vi "E4981_command.vi"(8 "error in (no error)":errorcluster, 10 "input":T1={"Frequency (1:1kHz)"=1, "Frequency Shift (2: 0%)"=2, "Range"=enum."1p"} {"Frequency Shift (2: 0%)" items=["-2%", "-1%", "0%", "1%", "2%"]; "Frequency (1:1kHz)" items=["120 Hz Frequency", "1 kHz Frequency", "1 MHz Frequency"]}, 11 "command":T3(ring)) -> (0 "error out":errorcluster, 1 "bin":i32, 3 "output":T2={"connectd"=TRUE, "CAP cab"=0.0, "DF  Cab"=0.0} {"CAP cab" format="%#_6p"})   [LabVIEW 2016]
uses:
  meter global.vi
  AOIFramwork/AOIFramework.lvlib
panel:
  in  "reset":bool
  # "CAP DF 電錶作業中"
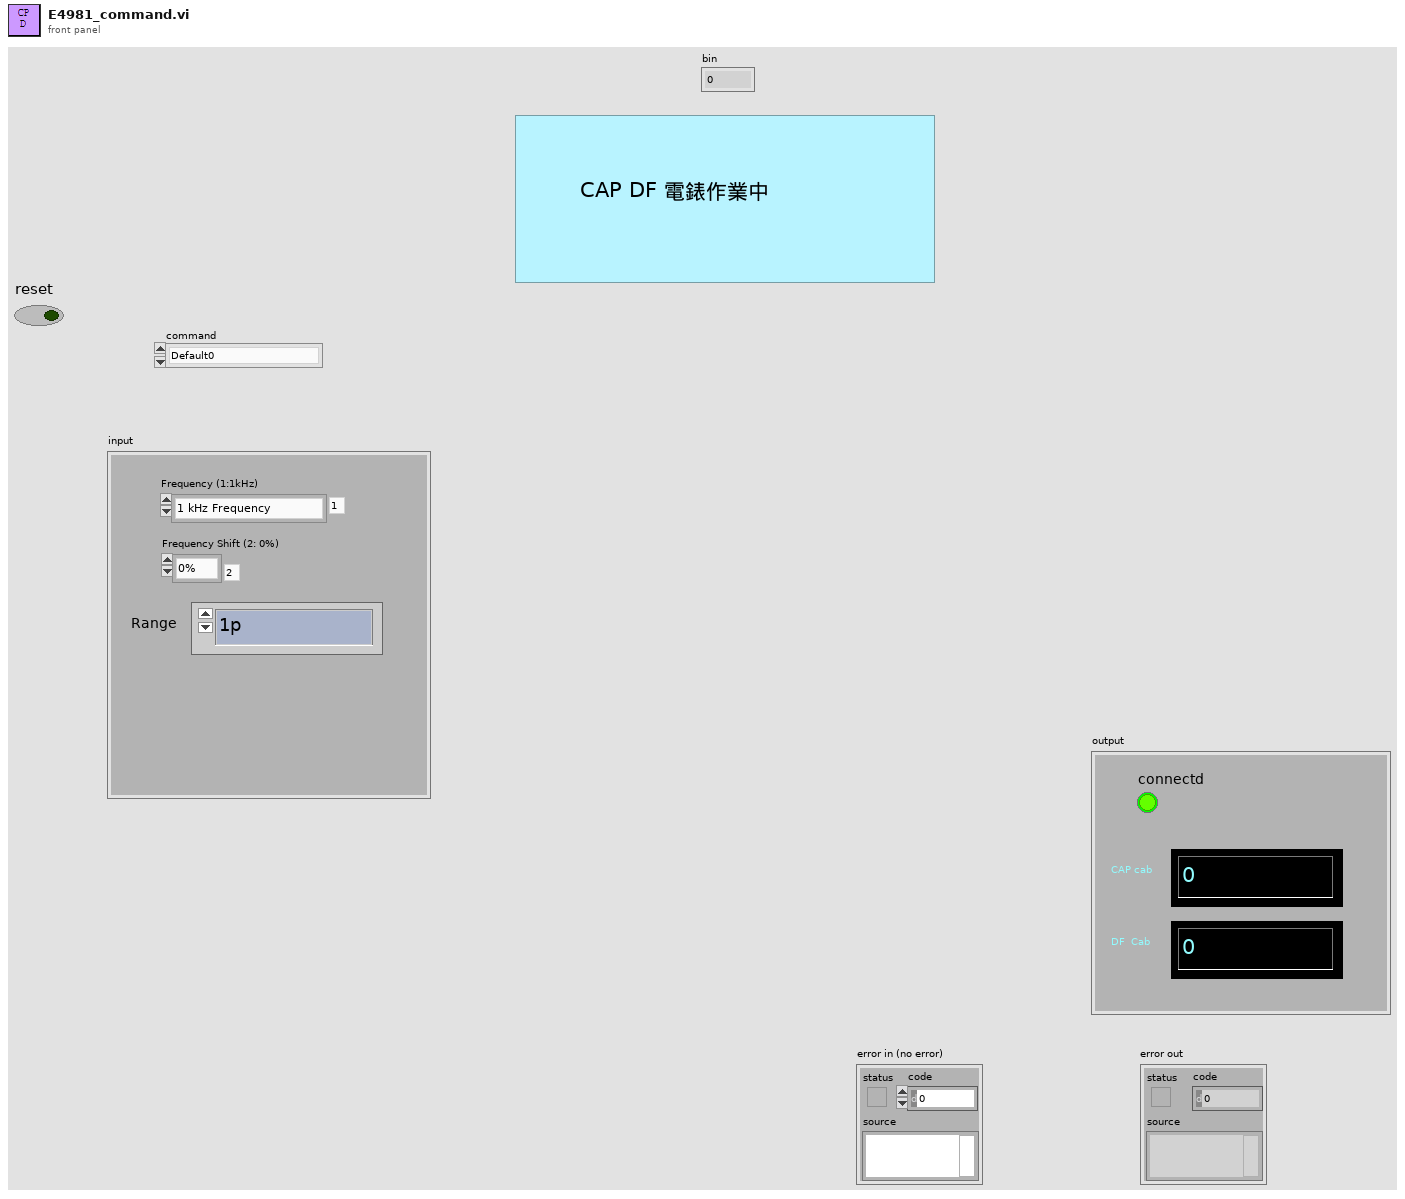
[diagram p1: front panel]
types:
  T1 = cluster{"Frequency (1:1kHz)":u16, "Frequency Shift (2: 0%)":u16, "Range":enum16{"1p", "2.2p", "4.7p", "10p", "22p", "47p", "100p", "220p", "470p", "1n", "2.2n", "4.7n", "10n", "22n", "47n", "100n", "220n", "470n", "1u", "2.2u", "4.7u", "10u", "22u", "47u", "100u", "220u", "470u", "1m", "AUTO", ""}}
  T2 = cluster{"connectd":bool, "CAP cab":dbl, "DF  Cab":dbl}
  T3 = enum16{"Default0", "checkconnect", "int", "changeFEQ", "changeRange", "trigger", "triggerauto"}
  T4 = enum16{"1p", "2.2p", "4.7p", "10p", "22p", "47p", "100p", "220p", "470p", "1n", "2.2n", "4.7n", "10n", "22n", "47n", "100n", "220n", "470n", "1u", "2.2u", "4.7u", "10u", "22u", "47u", "100u", "220u", "470u", "1m", "AUTO", ""}
  T5 = typedef "TypeDef_PNData.ctl" = cluster{"External Diameter":dbl, "Height":dbl, "Range":enum16{"1p", "2.2p", "4.7p", "10p", "22p", "47p", "100p", "220p", "470p", "1n", "2.2n", "4.7n", "10n", "22n", "47n", "100n", "220n", "470n", "1u", "2.2u", "4.7u", "10u", "22u", "47u", "100u", "220u", "470u", "1m", "AUTO", ""}, "DFmin":dbl, "Cap_num":dbl, "F":u16, "BIN3+":dbl, "BIN3- ":dbl, "BIN2+":dbl, "BIN2-":dbl, "BIN1+":dbl, "BIN1-":dbl, "Frequencies":enum16{"120HZ", "1K  HZ", "1M HZ"}, "DFmax":dbl, "Part_5":dbl, "Part_6":dbl, "Part_4":dbl, "Part_8":dbl, "Part_7":dbl, "Par_2":dbl, "part_1":enum16{"DC", "AC"}, "Part_9":dbl, "Part_18":dbl, "Part_15":dbl, "Part_13":dbl, "Part_14":dbl, "Part_16":dbl, "Internal Diameter":dbl, "Part_14 (IR Max)":dbl, "SCARA Place Offset":T6}
  T6 = typedef "MachineParTypeSCARA PlaceOffset.ctl" = cluster{"Buffer":cluster{"X":dbl, "Y":dbl, "Z":dbl}, "UNLD":cluster{"X":dbl, "Y":dbl, "Z":dbl}}
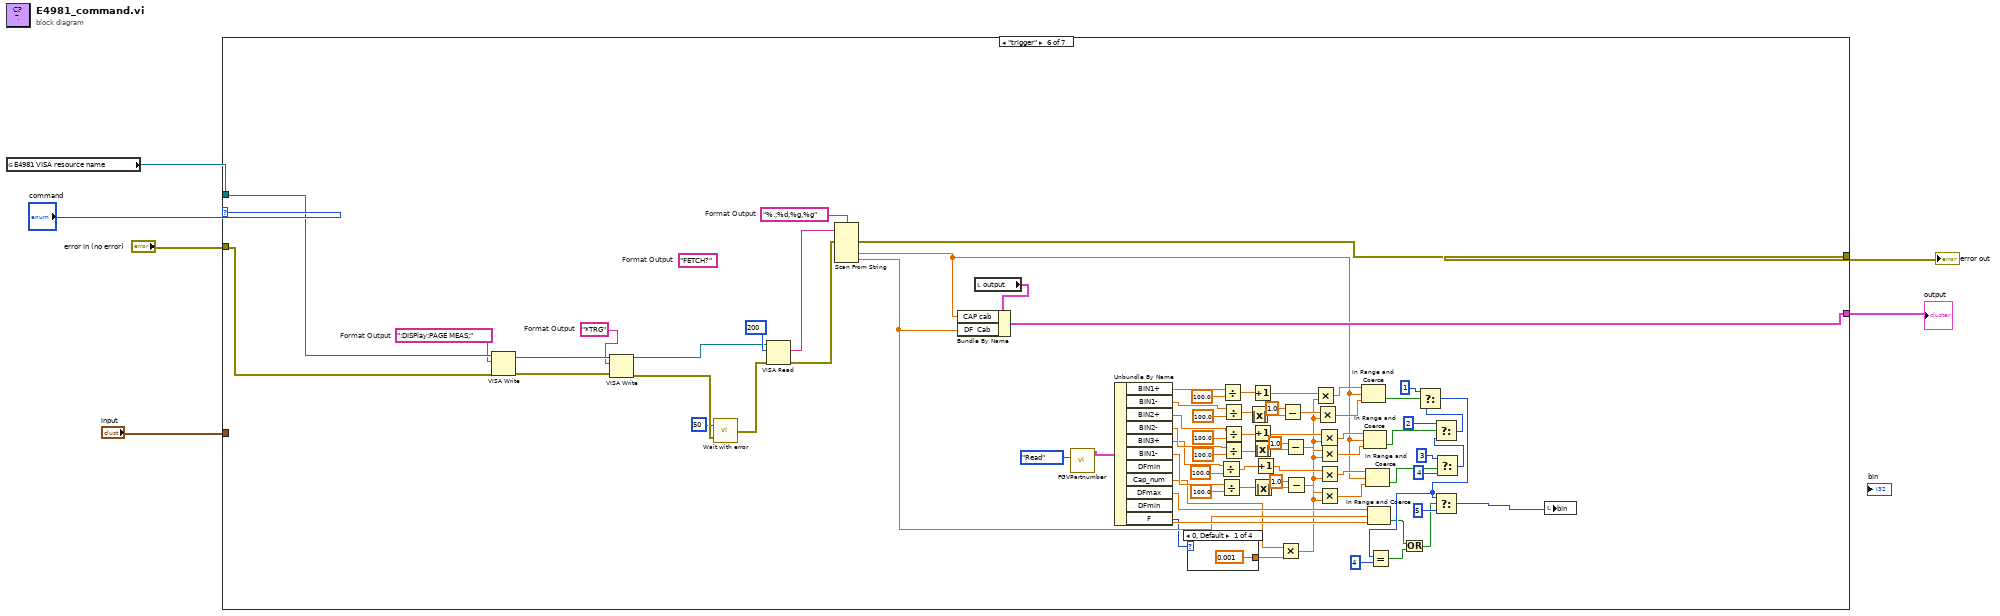
[diagram p0: block diagram]
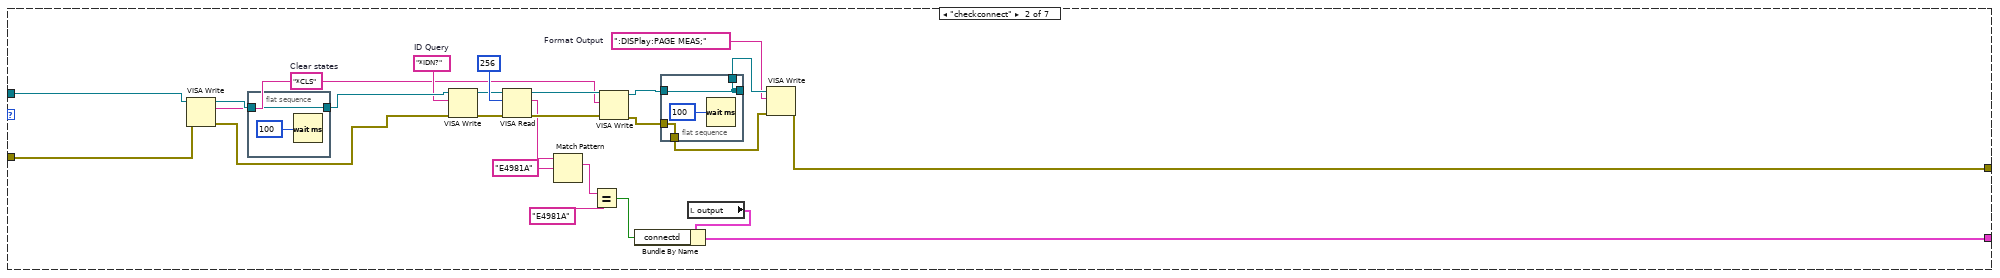
[diagram p3: hidden frame]
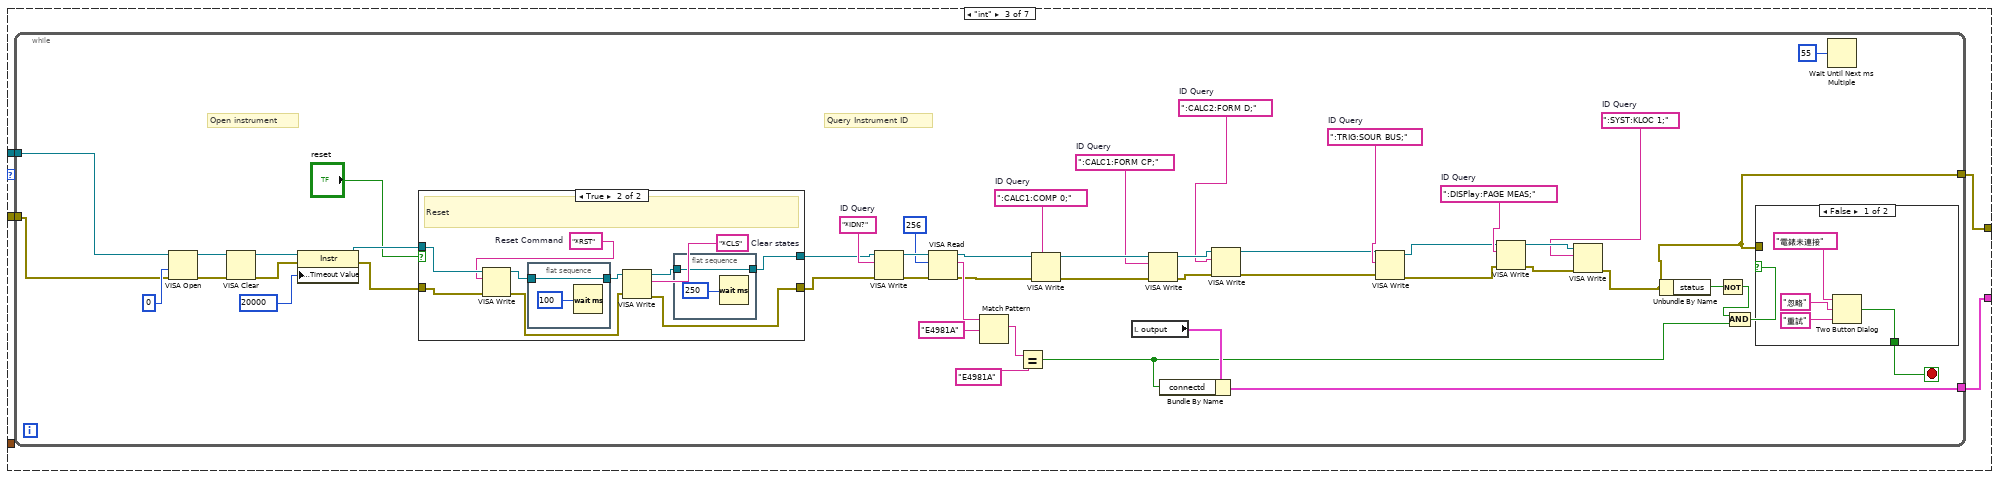
[diagram p4: hidden frame]
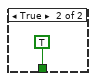
[diagram p6: hidden frame]
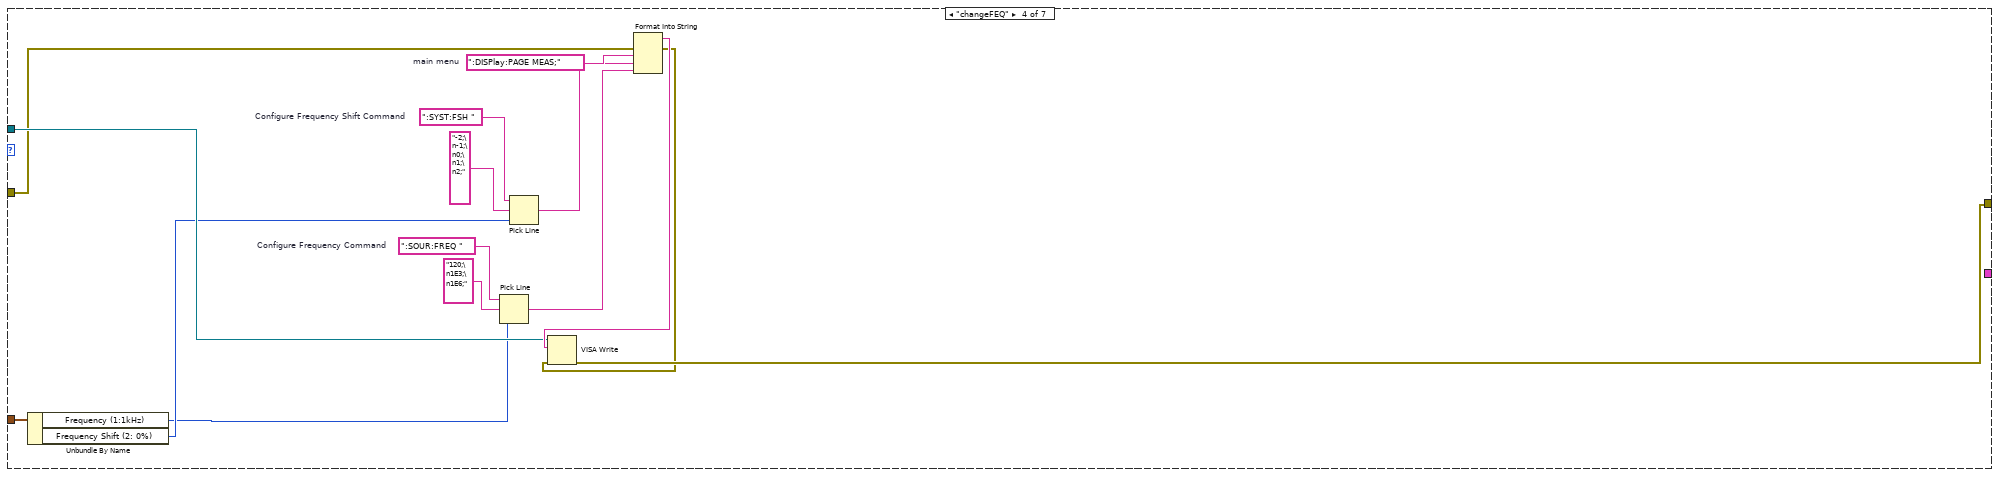
[diagram p7: hidden frame]
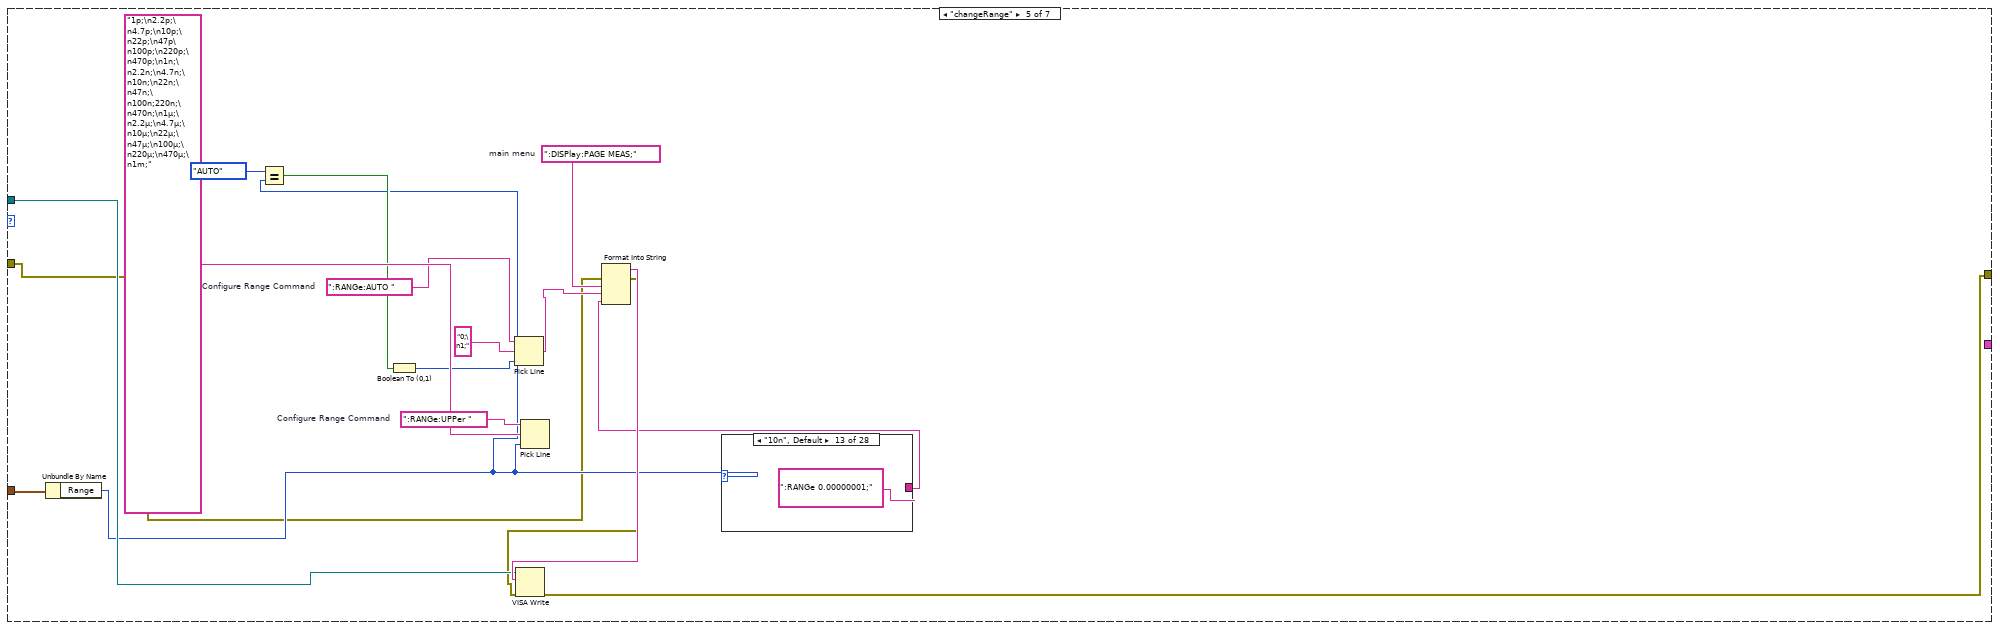
[diagram p8: hidden frame]
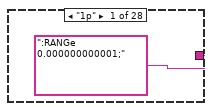
[diagram p9: hidden frame]
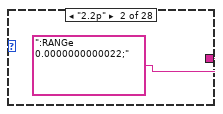
[diagram p10: hidden frame]
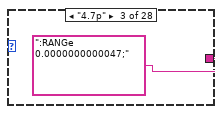
[diagram p11: hidden frame]
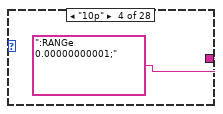
[diagram p12: hidden frame]
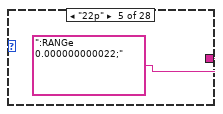
[diagram p13: hidden frame]
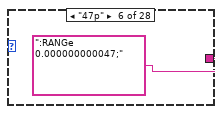
[diagram p14: hidden frame]
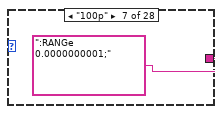
[diagram p15: hidden frame]
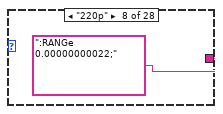
[diagram p16: hidden frame]
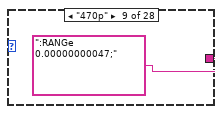
[diagram p17: hidden frame]
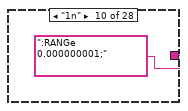
[diagram p18: hidden frame]
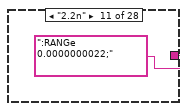
[diagram p19: hidden frame]
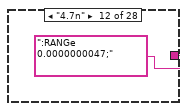
[diagram p20: hidden frame]
diagram:
  n1 = global read "meter global.vi" "E4981 VISA resource name"() -> (w4:refnum<visa-resource-name>)
  n2 = case shown="\"trigger\"" "command" {
    tunnel: "error in (no error)" -> [_ w13 w38 w111 w126 w240 w319]
    tunnel: [_ w12 w40 w115 w129 w235 w261] -> w5
    tunnel: w4 -> [_ w10 w39 w116 w130 w241 w320]
    tunnel: [_ w7 w37 _ _ w238 w317] -> w2
    tunnel: "input" -> [_ _ _ w114 w128 _ _]
    frame "Default0", Default {
    }
    frame "checkconnect" {
      w27 = ":DISPlay:PAGE MEAS;"  # Format Output
      w11 = "*CLS"  # Clear states
      w19 = "*IDN?"  # ID Query
      n3 = VISA Write(VISA resource name=w10, write buffer=w11, error in (no error)=w13) -> (VISA resource name out=w24:refnum<visa-resource-name>, error out=w23:errorcluster)  [unwired: 1 out]
      n4 = flat-sequence {
        tunnel: [w35] -> w22
        tunnel: w24 -> [w35]
        frame #0 {
          n5 = Wait (ms)(milliseconds to wait=u32 100) -> ()  [unwired: 1 out]
        }
      }
      n6 = VISA Write(VISA resource name=w22, write buffer=w19, error in (no error)=w23) -> (VISA resource name out=w15:refnum<visa-resource-name>, error out=w16:errorcluster)  [unwired: 1 out]
      n7 = VISA Read(VISA resource name=w15, byte count=u32 256, error in (no error)=w16) -> (VISA resource name out=w25:refnum<visa-resource-name>, read buffer=w14:string, error out=w26:errorcluster)  [unwired: 1 out]
      n8 = Match Pattern(string=w14, regular expression="E4981A") -> (match substring=w20:string)  [unwired: 1 in, 3 out]
      n9 = Equal?(x=w20, y="E4981A") -> (x = y?=w8:bool)
      n10 = VISA Write(VISA resource name=w25, write buffer=w11, error in (no error)=w26) -> (VISA resource name out=w28:refnum<visa-resource-name>, error out=w29:errorcluster)  [unwired: 1 out]
      n11 = flat-sequence {
        tunnel: [w32] -> _
        tunnel: w28 -> [w32]
        tunnel: w29 -> [w33]
        tunnel: [w33] -> w30
        tunnel: [w32] -> w31
        frame #0 {
          n12 = Wait (ms)(milliseconds to wait=u32 100) -> ()  [unwired: 1 out]
        }
      }
      n13 = local read "output"() -> (w9:T2)
      n14 = Bundle By Name(cluster=w9, "connectd"=w8) -> (w7:T2)
      n15 = VISA Write(VISA resource name=w31, write buffer=w27, error in (no error)=w30) -> (error out=w12:errorcluster)  [unwired: 2 out]
    }
    frame "int" {
      n16 = while {
        tunnel: [w46] -> w40
        tunnel: w39 -> [w45]
        tunnel: w38 -> [w44]
        tunnel: [w41] -> w37
        stop <- w73 stop-if-true
        w54 = ":TRIG:SOUR BUS;"  # ID Query
        w57 = ":SYST:KLOC 1;"  # ID Query
        w60 = ":DISPlay:PAGE MEAS;"  # ID Query
        w61 = ":CALC2:FORM D;"  # ID Query
        w62 = ":CALC1:FORM CP;"  # ID Query
        w71 = ":CALC1:COMP 0;"  # ID Query
        w77 = "*IDN?"  # ID Query
        # "Query Instrument ID"
        # "Open instrument"
        n17 = VISA Open(access mode=u32 0, error in (no error)=w44, VISA resource name=w45) -> (VISA resource name=w86:refnum<visa-resource-name>, error out=w85:errorcluster)  [unwired: 2 in]
        n18 = VISA Clear(VISA resource name=w86, error in (no error)=w85) -> (VISA resource name out=w84:refnum<visa-resource-name>, error out=w83:errorcluster)
        n19 = property class="Instr"(reference=w84, error in=w83, "General Settings:Timeout Value"=u32 20000) -> (reference out=w50:refnum<visa-resource-name>, error out=w48:errorcluster)
        n20 = case shown="True" "reset" {
          tunnel: [w90 w95] -> w51
          tunnel: w50 -> [w90 w100]
          tunnel: [w89 w93] -> w49
          tunnel: w48 -> [w89 w92]
          frame False {
          }
          frame True {
            w91 = "*CLS"  # Clear states
            w99 = "*RST"  # Reset Command
            # "Reset"
            n21 = VISA Write(VISA resource name=w100, write buffer=w99, error in (no error)=w92) -> (VISA resource name out=w97:refnum<visa-resource-name>, error out=w94:errorcluster)  [unwired: 1 out]
            n22 = flat-sequence {
              tunnel: [w103] -> w98
              tunnel: w97 -> [w103]
              frame #0 {
                n23 = Wait (ms)(milliseconds to wait=u32 100) -> ()  [unwired: 1 out]
              }
            }
            n24 = VISA Write(VISA resource name=w98, write buffer=w91, error in (no error)=w94) -> (VISA resource name out=w96:refnum<visa-resource-name>, error out=w93:errorcluster)  [unwired: 1 out]
            n25 = flat-sequence {
              tunnel: [w101] -> w95
              tunnel: w96 -> [w101]
              frame #0 {
                n26 = Wait (ms)(milliseconds to wait=u32 250) -> ()  [unwired: 1 out]
              }
            }
          }
        }
        n27 = VISA Write(VISA resource name=w51, write buffer=w77, error in (no error)=w49) -> (VISA resource name out=w81:refnum<visa-resource-name>, error out=w80:errorcluster)  [unwired: 1 out]
        n28 = VISA Read(VISA resource name=w81, byte count=u32 256, error in (no error)=w80) -> (VISA resource name out=w69:refnum<visa-resource-name>, read buffer=w82:string, error out=w70:errorcluster)  [unwired: 1 out]
        n29 = Match Pattern(string=w82, regular expression="E4981A") -> (match substring=w75:string)  [unwired: 1 in, 3 out]
        n30 = Equal?(x=w75, y="E4981A") -> (x = y?=w42:bool)
        n31 = VISA Write(VISA resource name=w69, write buffer=w71, error in (no error)=w70) -> (VISA resource name out=w66:refnum<visa-resource-name>, error out=w65:errorcluster)  [unwired: 1 out]
        n32 = local read "output"() -> (w43:T2)
        n33 = VISA Write(VISA resource name=w66, write buffer=w62, error in (no error)=w65) -> (VISA resource name out=w63:refnum<visa-resource-name>, error out=w64:errorcluster)  [unwired: 1 out]
        n34 = Bundle By Name(cluster=w43, "connectd"=w42) -> (w41:T2)
        n35 = VISA Write(VISA resource name=w63, write buffer=w61, error in (no error)=w64) -> (VISA resource name out=w53:refnum<visa-resource-name>, error out=w52:errorcluster)  [unwired: 1 out]
        n36 = VISA Write(VISA resource name=w53, write buffer=w54, error in (no error)=w52) -> (VISA resource name out=w56:refnum<visa-resource-name>, error out=w55:errorcluster)  [unwired: 1 out]
        n37 = VISA Write(VISA resource name=w56, write buffer=w60, error in (no error)=w55) -> (VISA resource name out=w58:refnum<visa-resource-name>, error out=w59:errorcluster)  [unwired: 1 out]
        n38 = VISA Write(VISA resource name=w58, write buffer=w57, error in (no error)=w59) -> (error out=w46:errorcluster)  [unwired: 2 out]
        n39 = Unbundle By Name(w46) -> ("status"=w68:bool)
        n40 = Not(x=w68) -> (.not. x?=w67:bool)
        n41 = And(x=w67, y=w42) -> (x .and. y?=w76:bool)
        n42 = case shown="False" w76 {
          tunnel: [w107 TRUE ("cancel 2")] -> w73
          tunnel: w46 -> [_ _]
          frame False {
            n43 = Two Button Dialog(message="電錶未連接", 1:"重試" ("T button name (\"OK\")"), 2:"忽略" ("F button name (\"Cancel\")")) -> (T button?=w107:bool)
          }
          frame True {
          }
        }
        n44 = Wait Until Next ms Multiple(millisecond multiple=u32 55) -> ()  [unwired: 1 out]
      }
    }
    frame "changeFEQ" {
      w120 = ":DISPlay:PAGE MEAS;"  # main menu
      w121 = ":SYST:FSH "  # Configure Frequency Shift Command
      w122 = ":SOUR:FREQ "  # Configure Frequency Command
      n45 = Unbundle By Name(w114) -> ("Frequency (1:1kHz)"=w112:u16, "Frequency Shift (2: 0%)"=w113:u16)
      n46 = Pick Line(string ("")=w122, multi-line string="120;\n1E3;\n1E6;", line index=w112) -> (output string=w118:string)
      n47 = Pick Line(string ("")=w121, multi-line string="-2;\n-1;\n0;\n1;\n2;", line index=w113) -> (output string=w119:string)
      n48 = Format Into String(error in=w111, w120, w119, w118) -> (resulting string=w117:string, error out=w110:errorcluster)  [unwired: 2 in]
      n49 = VISA Write(VISA resource name=w116, write buffer=w117, error in (no error)=w110) -> (error out=w115:errorcluster)  [unwired: 2 out]
    }
    frame "changeRange" {
      w139 = ":RANGe:UPPer "  # Configure Range Command
      w136 = ":RANGe:AUTO "  # Configure Range Command
      w141 = ":DISPlay:PAGE MEAS;"  # main menu
      n50 = Unbundle By Name(w128) -> ("Range"=w127:T4)
      n51 = Equal?(x=T4."AUTO", y=w127) -> (x = y?=w134:bool)
      n52 = Boolean To (0,1)(Boolean=w134) -> (0, 1=w133:i16)
      n53 = Pick Line(string ("")=w136, multi-line string="0;\n1;", line index=w133) -> (output string=w132:string)
      n54 = Pick Line(string ("")=w139, multi-line string="1p;\n2.2p;\n4.7p;\n10p;\n22p;\n47p\n100p;\n220p;\n470p;\n1n;\n2.2n;\n4.7n;\n10n;\n22n;\n47n;\n100n;220n;\n470n;\n1μ;\n2.2μ;\n4.7μ;\n10μ;\n22μ;\n47μ;\n100μ;\n220μ;\n470μ;\n1m;", line index=w127) -> ()  [unwired: 1 out]
      n55 = case shown="\"10n\", Default" w127 {
        tunnel: [":RANGe 0.000000000001;" ("Configure Range Command") ":RANGe 0.0000000000022;" ("Configure Range Command") ":RANGe 0.0000000000047;" ("Configure Range Command") ":RANGe 0.00000000001;" ("Configure Range Command") ":RANGe 0.000000000022;" ("Configure Range Command") ":RANGe 0.000000000047;" ("Configure Range Command") ":RANGe 0.0000000001;" ("Configure Range Command") ":RANGe 0.00000000022;" ("Configure Range Command") ":RANGe 0.00000000047;" ("Configure Range Command") ":RANGe 0.000000001;" ("Configure Range Command") ":RANGe 0.0000000022;" ("Configure Range Command") ":RANGe 0.0000000047;" ("Configure Range Command") ":RANGe 0.00000001;" ("Configure Range Command") ":RANGe 0.000000022;" ("Configure Range Command") ":RANGe 0.000000047;" ("Configure Range Command") ":RANGe 0.0000001;" ("Configure Range Command") ":RANGe 0.00000022;" ("Configure Range Command") ":RANGe 0.00000047;" ("Configure Range Command") ":RANGe 0.000001;" ("Configure Range Command") ":RANGe 0.0000022;" ("Configure Range Command") ":RANGe 0.0000047;" ("Configure Range Command") ":RANGe 0.00001;" ("Configure Range Command") ":RANGe 0.000022;" ("Configure Range Command") ":RANGe 0.000047;" ("Configure Range Command") ":RANGe 0.0001;" ("Configure Range Command") ":RANGe 0.00022;" ("Configure Range Command") ":RANGe 0.00047;" ("Configure Range Command") ":RANGe 0.001;" ("Configure Range Command")] -> w131
        frame "1p" {
        }
        frame "2.2p" {
        }
        frame "4.7p" {
        }
        frame "10p" {
        }
        frame "22p" {
        }
        frame "47p" {
        }
        frame "100p" {
        }
        frame "220p" {
        }
        frame "470p" {
        }
        frame "1n" {
        }
        frame "2.2n" {
        }
        frame "4.7n" {
        }
        frame "10n", Default {
        }
        frame "22n" {
        }
        frame "47n" {
        }
        frame "100n" {
        }
        frame "220n" {
        }
        frame "470n" {
        }
        frame "1u" {
        }
        frame "2.2u" {
        }
        frame "4.7u" {
        }
        frame "10u" {
        }
        frame "22u" {
        }
        frame "47u" {
        }
        frame "100u" {
        }
        frame "220u" {
        }
        frame "470u" {
        }
        frame "1m" {
        }
      }
      n56 = Format Into String(error in=w126, w141, w132, w131) -> (resulting string=w140:string, error out=w125:errorcluster)  [unwired: 2 in]
      n57 = VISA Write(VISA resource name=w130, write buffer=w140, error in (no error)=w125) -> (error out=w129:errorcluster)  [unwired: 2 out]
    }
    frame "trigger" {
      w237 = ":DISPlay:PAGE MEAS;"  # Format Output
      (unwired) "FETCH?"  # Format Output
      w242 = "*TRG"  # Format Output
      w246 = "%.;%d,%g,%g"  # Format Output
      n58 = VISA Write(VISA resource name=w241, write buffer=w237, error in (no error)=w240) -> (VISA resource name out=w243:refnum<visa-resource-name>, error out=w244:errorcluster)  [unwired: 1 out]
      n59 = VISA Write(VISA resource name=w243, write buffer=w242, error in (no error)=w244) -> (VISA resource name out=w245:refnum<visa-resource-name>, error out=w177:errorcluster)  [unwired: 1 out]
      n60 = call "Wait with error.vi"("error in (no error)"=w177, "milliseconds to wait"=u32 50) -> ("error out"=w176:errorcluster)
      n61 = VISA Read(VISA resource name=w245, byte count=u32 200, error in (no error)=w176) -> (read buffer=w247:string, error out=w236:errorcluster)  [unwired: 2 out]
      n62 = Scan From String(format string=w246, input string=w247, error in=w236) -> (error out=w235:errorcluster, output 2=w183:dbl, output 3=w182:dbl)  [unwired: 5 in, 2 out]
      n63 = local read "output"() -> (w239:T2)
      n64 = Bundle By Name(cluster=w239, "CAP cab"=w183, "DF  Cab"=w182) -> (w238:T2)
      n65 = call "FGVPartnumber.vi"("Enum"=enum16{"Write", "Read"}."Read") -> ("UnitParamiterCluster out"=w233:T5)  [unwired: 9 in, 1 out]
      n66 = Unbundle By Name(w233) -> ("BIN1+"=w232:dbl, "BIN1-"=w229:dbl, "BIN2+"=w227:dbl, "BIN2-"=w225:dbl, "BIN3+"=w223:dbl, "BIN1-"=w221:dbl, "Cap_num"=w179:dbl, "DFmax"=w196:dbl, "DFmin"=w195:dbl, "F"=w181:u16)  [unwired: 1 out]
      n67 = case shown="0, Default" w181 {
        tunnel: [0.001 1e-06 1e-09 1e-12] -> w180
        frame 0, Default {
        }
        frame 1 {
        }
        frame 2 {
        }
        frame 3 {
        }
      }
      n68 = Divide(x=w223, y=100.0) -> (x/y=w209:dbl)
      n69 = Divide(x=w221, y=100.0) -> (x/y=w211:dbl)
      n70 = Divide(x=w232, y=100.0) -> (x/y=w220:dbl)
      n71 = Divide(x=w229, y=100.0) -> (x/y=w219:dbl)
      n72 = Divide(x=w227, y=100.0) -> (x/y=w210:dbl)
      n73 = Divide(x=w225, y=100.0) -> (x/y=w214:dbl)
      n74 = Absolute Value(x=w219) -> (abs(x)=w218:dbl)
      n75 = Increment(x=w220) -> (x+1=w208:dbl)
      n76 = Increment(x=w210) -> (x+1=w206:dbl)
      n77 = Absolute Value(x=w214) -> (abs(x)=w215:dbl)
      n78 = Absolute Value(x=w211) -> (abs(x)=w213:dbl)
      n79 = Increment(x=w209) -> (x+1=w204:dbl)
      n80 = Multiply(x=w179, y=w180) -> (x*y=w178:dbl)
      n81 = Subtract(x=1.0, y=w218) -> (x-y=w207:dbl)
      n82 = Subtract(x=1.0, y=w215) -> (x-y=w205:dbl)
      n83 = Subtract(x=1.0, y=w213) -> (x-y=w203:dbl)
      n84 = Multiply(x=w208, y=w178) -> (x*y=w202:dbl)
      n85 = Multiply(x=w207, y=w178) -> (x*y=w201:dbl)
      n86 = Multiply(x=w206, y=w178) -> (x*y=w200:dbl)
      n87 = Multiply(x=w205, y=w178) -> (x*y=w199:dbl)
      n88 = Multiply(x=w204, y=w178) -> (x*y=w198:dbl)
      n89 = Multiply(x=w203, y=w178) -> (x*y=w197:dbl)
      n90 = In Range and Coerce(upper limit=w202, x=w183, lower limit=w201) -> (In Range?=w194:bool)  [unwired: 1 out]
      n91 = In Range and Coerce(upper limit=w200, x=w183, lower limit=w199) -> (In Range?=w187:bool)  [unwired: 1 out]
      n92 = In Range and Coerce(upper limit=w198, x=w183, lower limit=w197) -> (In Range?=w189:bool)  [unwired: 1 out]
      n93 = In Range and Coerce(upper limit=w196, x=w182, lower limit=w195) -> (In Range?=w171:bool)  [unwired: 1 out]
      n94 = Select(t=3, s=w189, f=4) -> (s? t:f=w188:i32)
      n95 = Select(t=2, s=w187, f=w188) -> (s? t:f=w186:i32)
      n96 = Select(t=1, s=w194, f=w186) -> (s? t:f=w174:i32)
      n97 = Equal?(x=w174, y=4) -> (x = y?=w172:bool)
      n98 = Or(x=w171, y=w172) -> (x .or. y?=w170:bool)
      n99 = Select(t=w174, s=w170, f=5) -> (s? t:f=w184:i32)
      n100 = local write "bin"(w184) -> ()
    }
    frame "triggerauto" {
      w316 = enum16{"Write", "Read"}."Read"  # Enum
      (unwired) "FETCH?"  # Format Output
      w321 = "*TRG"  # Format Output
      w325 = "%.;%d,%g,%g"  # Format Output
      n101 = disable-structure shown="Disabled" {
        disable-tunnel: [w336 w337] -> w323
        disable-tunnel: [w335 w338] -> w322
        disable-tunnel: w320 -> [w334 w338]
        disable-tunnel: w319 -> [w333 w337]
        frame Disabled {
          w332 = ":DISPlay:PAGE MEAS;"  # Format Output
          n102 = VISA Write(VISA resource name=w334, write buffer=w332, error in (no error)=w333) -> (VISA resource name out=w335:refnum<visa-resource-name>, error out=w336:errorcluster)  [unwired: 1 out]
        }
        frame Enabled {
        }
      }
      n103 = VISA Write(VISA resource name=w322, write buffer=w321, error in (no error)=w323) -> (VISA resource name out=w324:refnum<visa-resource-name>, error out=w255:errorcluster)  [unwired: 1 out]
      n104 = call "Wait with error.vi"("error in (no error)"=w255, "milliseconds to wait"=u32 50) -> ("error out"=w254:errorcluster)
      n105 = VISA Read(VISA resource name=w324, byte count=u32 200, error in (no error)=w254) -> (read buffer=w326:string, error out=w262:errorcluster)  [unwired: 2 out]
      n106 = Scan From String(format string=w325, input string=w326, error in=w262) -> (error out=w261:errorcluster, output 2=w266:dbl, output 3=w265:dbl)  [unwired: 5 in, 2 out]
      n107 = local read "output"() -> (w318:T2)
      n108 = Bundle By Name(cluster=w318, "CAP cab"=w266, "DF  Cab"=w265) -> (w317:T2)
      n109 = call "FGVPartnumber.vi"("Enum"=w316) -> ("UnitParamiterCluster out"=w315:T5)  [unwired: 9 in, 1 out]
      n110 = Unbundle By Name(w315) -> ("BIN1+"=w314:dbl, "BIN1-"=w311:dbl, "BIN2+"=w309:dbl, "BIN2-"=w307:dbl, "BIN3+"=w305:dbl, "BIN1-"=w303:dbl, "Cap_num"=w257:dbl, "DFmax"=w278:dbl, "DFmin"=w277:dbl, "F"=w258:u16)  [unwired: 1 out]
      n111 = Divide(x=w305, y=100.0) -> (x/y=w291:dbl)
      n112 = Divide(x=w303, y=100.0) -> (x/y=w293:dbl)
      n113 = Divide(x=w314, y=100.0) -> (x/y=w302:dbl)
      n114 = Divide(x=w311, y=100.0) -> (x/y=w301:dbl)
      n115 = Divide(x=w309, y=100.0) -> (x/y=w292:dbl)
      n116 = Divide(x=w307, y=100.0) -> (x/y=w296:dbl)
      n117 = case shown="0, Default" w258 {
        tunnel: [0.001 1e-06 1e-09 1e-12] -> w259
        frame 0, Default {
        }
        frame 1 {
        }
        frame 2 {
        }
        frame 3 {
        }
      }
      n118 = Absolute Value(x=w301) -> (abs(x)=w300:dbl)
      n119 = Increment(x=w302) -> (x+1=w290:dbl)
      n120 = Increment(x=w292) -> (x+1=w288:dbl)
      n121 = Absolute Value(x=w296) -> (abs(x)=w297:dbl)
      n122 = Absolute Value(x=w293) -> (abs(x)=w295:dbl)
      n123 = Increment(x=w291) -> (x+1=w286:dbl)
      n124 = Subtract(x=1.0, y=w300) -> (x-y=w289:dbl)
      n125 = Subtract(x=1.0, y=w297) -> (x-y=w287:dbl)
      n126 = Subtract(x=1.0, y=w295) -> (x-y=w285:dbl)
      n127 = Multiply(x=w257, y=w259) -> (x*y=w256:dbl)
      n128 = Multiply(x=w290, y=w256) -> (x*y=w284:dbl)
      n129 = Multiply(x=w289, y=w256) -> (x*y=w283:dbl)
      n130 = Multiply(x=w288, y=w256) -> (x*y=w282:dbl)
      n131 = Multiply(x=w287, y=w256) -> (x*y=w281:dbl)
      n132 = Multiply(x=w286, y=w256) -> (x*y=w280:dbl)
      n133 = Multiply(x=w285, y=w256) -> (x*y=w279:dbl)
      n134 = In Range and Coerce(upper limit=w284, x=w266, lower limit=w283) -> (In Range?=w276:bool)  [unwired: 1 out]
      n135 = In Range and Coerce(upper limit=w282, x=w266, lower limit=w281) -> (In Range?=w268:bool)  [unwired: 1 out]
      n136 = In Range and Coerce(upper limit=w280, x=w266, lower limit=w279) -> (In Range?=w270:bool)  [unwired: 1 out]
      n137 = In Range and Coerce(upper limit=w278, x=w265, lower limit=w277) -> (In Range?=w271:bool)  [unwired: 1 out]
      n138 = Select(t=3, s=w270, f=4) -> (s? t:f=w269:i32)
      n139 = Select(t=2, s=w268, f=w269) -> (s? t:f=w267:i32)
      n140 = Select(t=1, s=w276, f=w267) -> (s? t:f=w263:i32)
      n141 = Select(t=w263, s=w271, f=5) -> (s? t:f=w260:i32)
      n142 = local write "bin"(w260) -> ()
    }
  }
  "error out" <- w5
  "output" <- w2
